vi "AdaptToInputs.vi"(0 "XRef":T13, 1 "Term Types":T10, 2 "State In":T1 {"BlockNodeState"."Draw Style" items=["FunctionBlock", "ExpressVI", "Variable", "Elemental I/O", "32x32 Icon", "FunctionBlockCompact"]; "BlockNodeState"."Terminal Data"."Terminal Flags" format="%.0b"}) -> (14 "Reply":T8, 15 "State Out":T1 {"BlockNodeState"."Draw Style" items=["FunctionBlock", "ExpressVI", "Variable", "Elemental I/O", "32x32 Icon", "FunctionBlockCompact"]; "BlockNodeState"."Terminal Data"."Terminal Flags" format="%.0b"})   [LabVIEW 2017, in "Set DDT Attributes.lvlib" / "Set DDT Properties.xnode"]
uses:
  <vilib>/express/express signal manip/GetorSetDDTAttributes/Set DDT Attributes/Set DDT Properties.xnode
  <vilib>/XNodeSupport/XNodeXNodeRef.ctl
  <vilib>/XNodeSupport/XNodeTermTypeIDPairs.ctl
  <vilib>/XNodeSupport/XNodeTermTypeIDPair.ctl
  <vilib>/XNodeSupport/XNodeType.ctl
  <vilib>/XNodeSupport/XNodeString.ctl
  <vilib>/express/express signal manip/GetorSetDDTAttributes/Set DDT Attributes/State.ctl
  <vilib>/BlockNodeSupport/BlockNodeState.ctl
  <vilib>/BlockNodeSupport/TerminalData.ctl
  <vilib>/picture/picture.llb/imagedata.ctl
  <vilib>/express/express signal manip/GetorSetDDTAttributes/Shared VIs/Attributes data.ctl
  <vilib>/express/express signal manip/GetorSetDDTAttributes/Shared VIs/Input.ctl
  <vilib>/express/express signal manip/GetorSetDDTAttributes/Shared VIs/Attributes name.ctl
  <vilib>/XNodeSupport/XNodeStringArray.ctl
  <vilib>/express/express signal manip/GetorSetDDTAttributes/Shared VIs/GetSetShared.lvlib
  <vilib>/XNodeSupport/NI_XNodeSupport.lvlib
  <vilib>/express/express signal manip/GetorSetDDTAttributes/Set DDT Attributes/Set DDT Attributes.lvlib
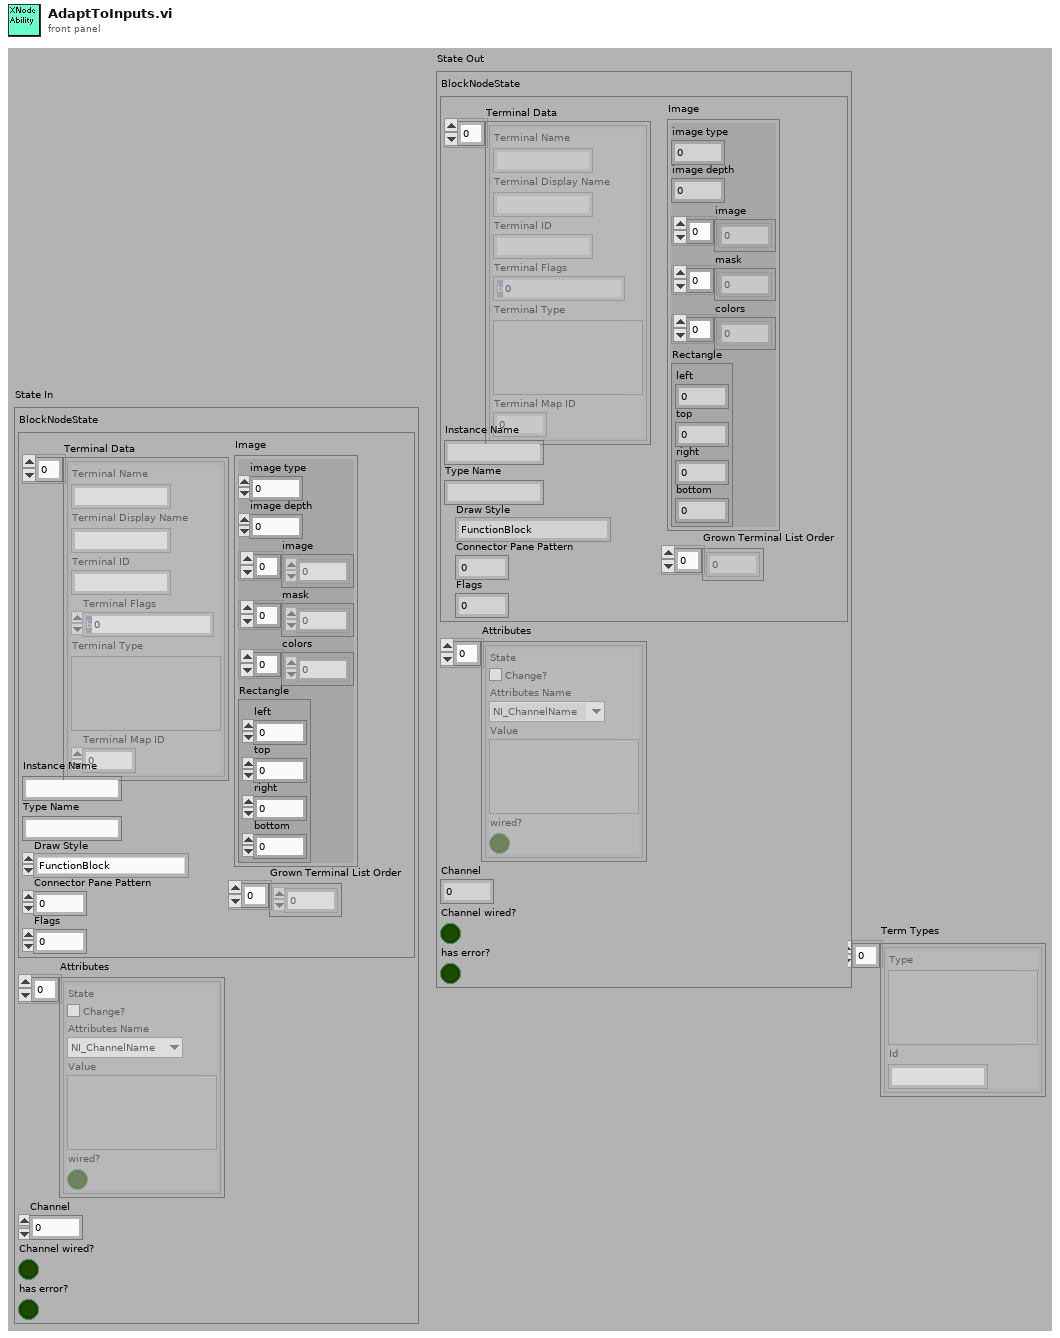
[diagram p1: front panel]
types:
  T1 = typedef "Set DDT Attributes.lvlib/Set DDT Properties.xnode/State.ctl" = cluster{"BlockNodeState":T2, "Attributes":T5[], "Channel":u32, "Channel wired?":bool, "has error?":bool}
  T2 = typedef "BlockNodeState.ctl" = cluster{"Terminal Data":T3[], "Instance Name":string, "Type Name":string, "Draw Style":i32, "Connector Pane Pattern":i32, "Flags":i32, "Grown Terminal List Order":i32[], "Image":T4}
  T3 = typedef "TerminalData.ctl" = cluster{"Terminal Name":string, "Terminal Display Name":string, "Terminal ID":string, "Terminal Flags":i32, "Terminal Type":variant, "Terminal Map ID":i32}
  T4 = typedef "imagedata.ctl" = cluster{"image type":i32, "image depth":i32, "image":u8[], "mask":u8[], "colors":u32[], "Rectangle":cluster{"left":i16, "top":i16, "right":i16, "bottom":i16}}
  T5 = typedef "GetSetShared.lvlib/Attributes data.ctl" = cluster{"State":T6, "Attributes Name":T7, "Value":variant, "wired?":bool}
  T6 = typedef "GetSetShared.lvlib/Input.ctl" = bool
  T7 = typedef "GetSetShared.lvlib/Attributes name.ctl" = enum16{"NI_ChannelName", "NI_ExpIsRelativeTime", "NI_ExpTimeStamp", "NI_ExpStartTimeStamp", "NI_ExpXDimension", "NI_UnitDescription"}
  T8 = typedef "NI_XNodeSupport.lvlib/XNodeStringArray.ctl" = T9[]
  T9 = typedef "NI_XNodeSupport.lvlib/XNodeString.ctl" = string
  T10 = typedef "NI_XNodeSupport.lvlib/XNodeTermTypeIDPairs.ctl" = T11[]
  T11 = typedef "NI_XNodeSupport.lvlib/XNodeTermTypeIDPair.ctl" = cluster{"Type":T12, "Id":T9}
  T12 = typedef "NI_XNodeSupport.lvlib/XNodeType.ctl" = variant
  T13 = typedef "NI_XNodeSupport.lvlib/XNodeXNodeRef.ctl" = refnum<vi>
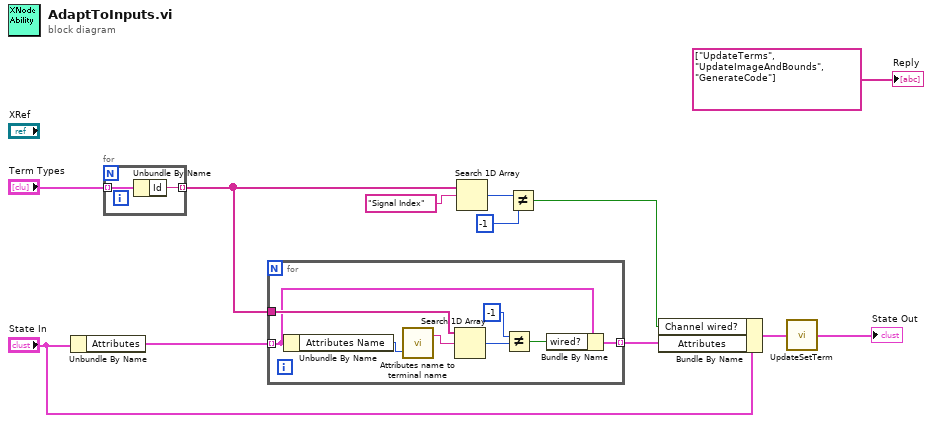
[diagram p0: block diagram]
diagram:
  n1 = Unbundle By Name("State In") -> ("Attributes"=w6:T5[])
  n2 = for {
    tunnel: "Term Types" -> [w14] mode=indexing
    tunnel: [w13] -> w7 mode=indexing
    n3 = Unbundle By Name(w14) -> ("Id"=w13:T9)
  }
  n4 = for {
    tunnel: w7 -> [w21]
    tunnel: w6 -> [w17] mode=indexing
    tunnel: [w16] -> w5 mode=indexing
    n5 = Unbundle By Name(w17) -> ("Attributes Name"=w22:T7)
    n6 = call <vilib>:"Attributes name to terminal name.vi"("Attributes Name"=w22) -> ("Terminal ID"=w15:string)  [unwired: 2 out]
    n7 = Search 1D Array(1D array=w21, element=w15) -> (index of element=w20:i32)  [unwired: 1 out]
    n8 = Not Equal?(x=-1, y=w20) -> (x != y?=w18:bool)
    n9 = Bundle By Name(cluster=w17, "wired?"=w18) -> (w16:T5)
  }
  n10 = Search 1D Array(1D array=w7, element=T9 "Signal Index") -> (index of element=w10:i32)  [unwired: 1 out]
  n11 = Not Equal?(x=w10, y=-1) -> (x != y?=w8:bool)
  n12 = Bundle By Name(cluster="State In", "Channel wired?"=w8, "Attributes"=w5) -> (w2:T1)
  n13 = call <vilib>:"UpdateSetTerm.vi"("State In"=w2) -> ("State Out"=→"State Out":T1)  [unwired: 2 out]
  "Reply" <- string[] ["UpdateTerms", "UpdateImageAndBounds", "GenerateCode"]
